vi "Execute.vi"(8 "error in (no error)":errorcluster, 10 "System In":refnum<class "abs_System.lvclass">, 11 "Node in":refnum<class "Wait.lvclass">) -> (0 "error out":errorcluster, 1 "Status":T1, 2 "System Out":refnum<class "abs_System.lvclass">, 3 "Node out":refnum<class "Wait.lvclass">)   [LabVIEW 2021, in "BT.lvlib" / "Wait.lvclass"]
uses:
  Wait.lvclass
  abs_Node/Status.ctl
  abs_System/abs_System.lvclass
  Wait.lvclass/Wait.ctl
  Properties/Read Time (ms).vi
  abs_Leaf/abs_Leaf.lvclass
  abs_Node/abs_Node.lvclass
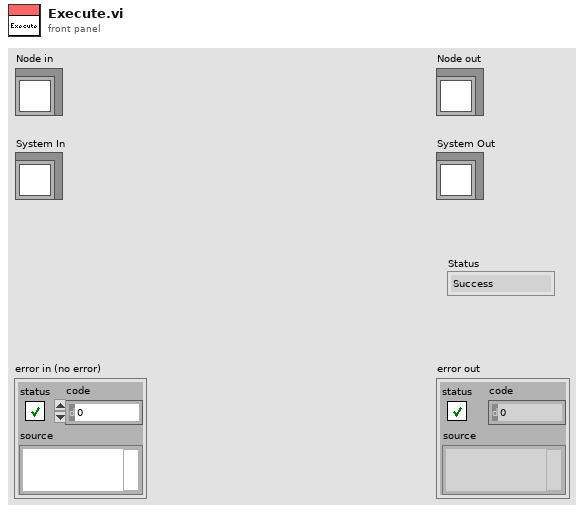
[diagram p1: front panel]
types:
  T1 = typedef "BT.lvlib/abs_Node.lvclass/Status.ctl" = enum16{"Success", "Failure", "Running"}
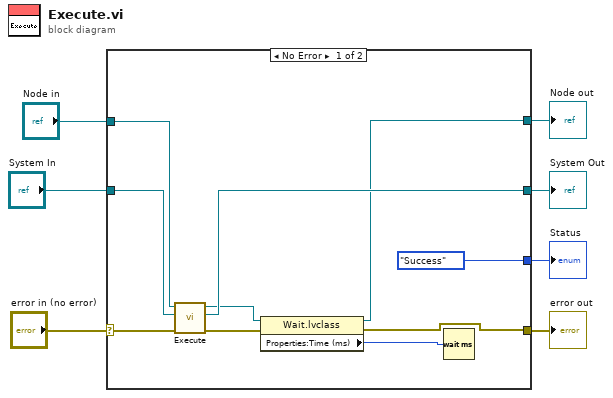
[diagram p0: block diagram]
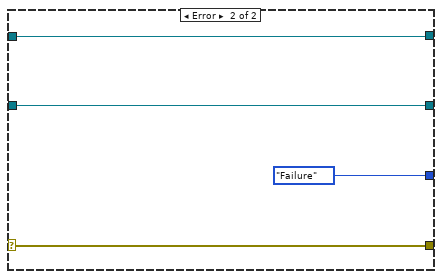
[diagram p2: hidden frame]
diagram:
  n1 = case shown="No Error" "error in (no error)" {
    selector: "error in (no error)" -> [w16 w19]
    tunnel: [w17 w20] -> w7
    tunnel: [w10 w21] -> w6
    tunnel: "System In" -> [w15 w20]
    tunnel: "Node in" -> [w14 w21]
    tunnel: [Status."Success" ("Status") Status."Failure" ("Status")] -> w2
    tunnel: [w8 w19] -> w1
    frame No Error {
      n2 = call-parent "Execute.vi"("error in (no error)"=w16, "System In"=w15, "Node in"=w14) -> ("error out"=w12:errorcluster, "System Out"=w17:refnum<class "abs_System.lvclass">, "Node out"=w11:refnum<class "Wait.lvclass">)  [unwired: 5 in, 1 out]
      n3 = property class="Wait.lvclass"(reference=w11, error in=w12) -> (reference out=w10:refnum<class "Wait.lvclass">, error out=w8:errorcluster, "Properties:Time (ms)"=w9:u32)
      n4 = Wait (ms)(milliseconds to wait=w9) -> ()  [unwired: 1 out]
    }
    frame Error {
    }
  }
  "error out" <- w1
  "Node out" <- w6
  "Status" <- w2
  "System Out" <- w7
